vi "Read Zones.vi"(8 "error in (no error)":errorcluster, 11 "StandardAttackPlay in":refnum<class "StandardAttackPlay.lvclass">) -> (0 "error out":errorcluster, 2 "Zones":refnum<class "Zone.lvclass">[](array[class]), 3 "StandardAttackPlay out":refnum<class "StandardAttackPlay.lvclass">)   [LabVIEW 2023, in "StandardAttackPlay.lvclass"]
uses:
  StandardAttackPlay.lvclass
  Zone_class/Zone.lvclass
  StandardAttackPlay.lvclass/StandardAttackPlay.ctl
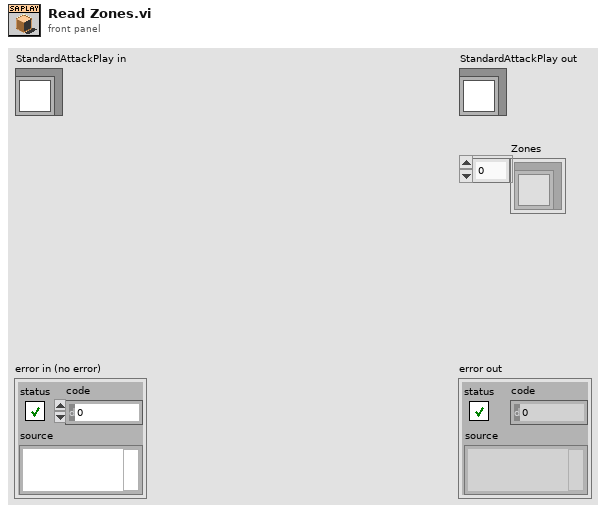
[diagram p1: front panel]
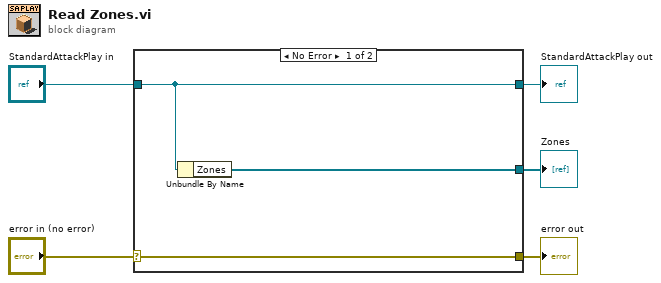
[diagram p0: block diagram]
diagram:
  n1 = case shown="No Error" "error in (no error)" {
    selector: "error in (no error)" -> [w8 w9]
    tunnel: [w8 w9] -> w4
    tunnel: [w7 w10] -> w2
    tunnel: "StandardAttackPlay in" -> [w7 w10]
    tunnel: [w6 _] -> w1
    frame No Error {
      n2 = Unbundle By Name(w7) -> ("Zones"=w6:refnum<class "Zone.lvclass">[])
    }
    frame Error {
    }
  }
  "error out" <- w4
  "StandardAttackPlay out" <- w2
  "Zones" <- w1
